vi "ReadDriveEncoder.vi"() -> ()   [LabVIEW 2012]
uses:
  Robot Global Data.vi
panel:
  out "EncoderR Alarm Status":string
  out "DistanceR (in)":dbl
  out "RevolutionsR":dbl
  out "Current angleR (deg)":dbl(knob) scale=0.0..360.0
  out "EncoderR Rate (deg/sec)":dbl
  out "EncoderR Direction":string
  in  "Reset EncoderR?":bool
  out "EncoderL Direction":string
  out "EncoderL Alarm Status":string
  in  "Reset EncoderL?":bool
  out "EncoderL Rate (deg/sec)":dbl
  out "RevolutionsL":dbl
  out "DistanceL (in)":dbl
  out "Current angleL (deg)":dbl(knob) scale=0.0..360.0
  out "error out":errorcluster
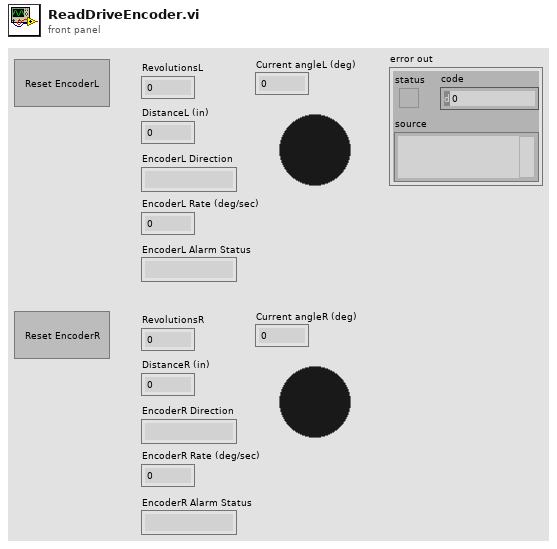
[diagram p1: front panel]
types:
  T1 = typedef "WPI_EncoderDevRef.ctl" = cluster{"DevStatus":errorcluster, "EncoderIndex":T2, "CounterIndex":T3, "DistancePerCount":dbl, "Decoding Type":T4}
  T2 = typedef "FPGA_EncoderIdx.ctl" = enum8{"Enc 0", "Enc 1", "Enc 2", "Enc 3", "Invalid"}
  T3 = typedef "FPGA_CounterCtrSystemIndex.ctl" = enum8{"Ctr 0", "Ctr 1", "Ctr 2", "Ctr 3", "Ctr 4", "Ctr 5", "Ctr 6", "Ctr 7", "Invalid"}
  T4 = typedef "WPI_EncoderType.ctl" = enum16{"1x", "2x", "4x"}
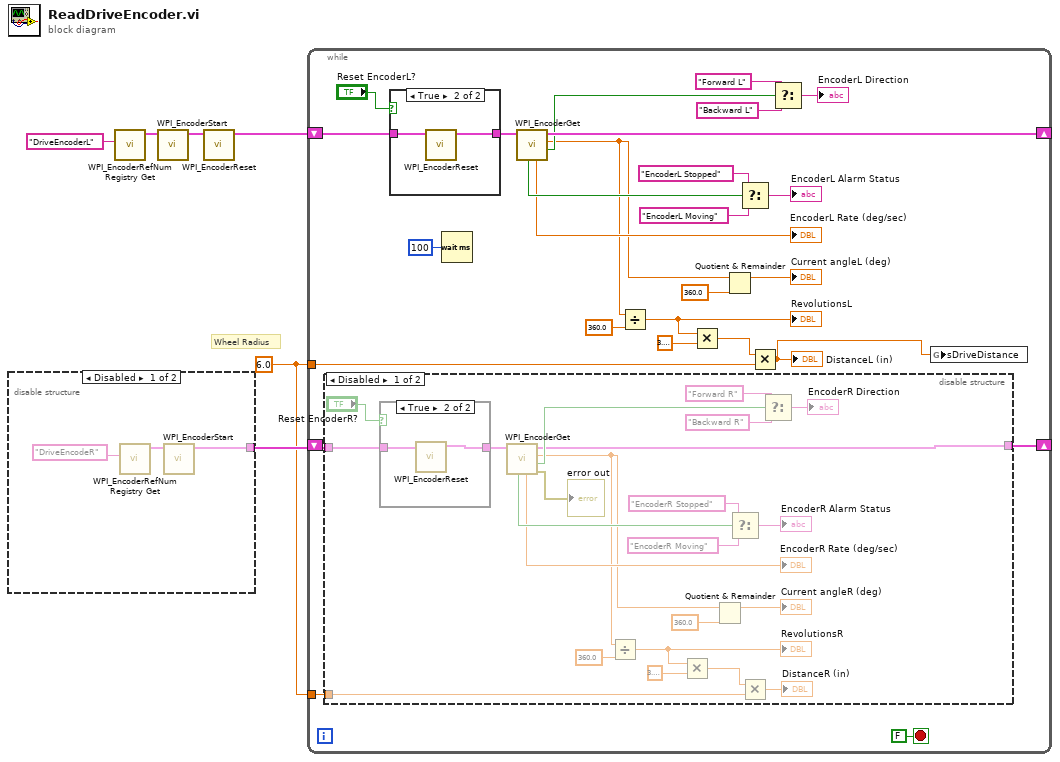
[diagram p0: block diagram]
diagram:
  w2 = 6.0
  # "Wheel Radius"
  n1 = disable-structure shown="Disabled" {
    disable-tunnel: [w7 _] -> w3
    frame Disabled {
      n2 = call <vilib>:"WPI_EncoderRefNum Registry Get.vi"("refnum name"="DriveEncodeR") -> ("EncoderDevRef"=w9:T1)  [unwired: 9 in, 1 out]
      n3 = call <vilib>:"WPI_EncoderStart.vi"("EncoderDevRef"=w9) -> ("EncoderDevRef"=w7:T1)  [unwired: 1 in, 9 out]
    }
    frame Enabled {
    }
  }
  n4 = call <vilib>:"WPI_EncoderRefNum Registry Get.vi"("refnum name"="DriveEncoderL") -> ("EncoderDevRef"=w6:T1)  [unwired: 9 in, 1 out]
  n5 = call <vilib>:"WPI_EncoderStart.vi"("EncoderDevRef"=w6) -> ("EncoderDevRef"=w5:T1)  [unwired: 1 in, 9 out]
  n6 = call <vilib>:"WPI_EncoderReset.vi"("EncoderDevRef"=w5) -> ("EncoderDevRef"=w1:T1)  [unwired: 1 in, 9 out]
  n7 = while {
    shift-right: [w32] -> _
    shift-left: w1 -> [w34]
    tunnel: w2 -> [w16]
    shift-right: [w14] -> _
    shift-left: w3 -> [w13]
    tunnel: w2 -> [w12]
    stop <- FALSE stop-if-true
    n8 = disable-structure shown="Disabled" {
      disable-tunnel: [w41 _] -> w14
      disable-tunnel: w13 -> [w40 _]
      disable-tunnel: w12 -> [w38 _]
      frame Disabled {
        n9 = case shown="True" "Reset EncoderR?" {
          tunnel: [w60 w62] -> w58
          tunnel: w40 -> [w60 w61]
          frame False {
          }
          frame True {
            n10 = call <vilib>:"WPI_EncoderReset.vi"("EncoderDevRef"=w61) -> ("EncoderDevRef"=w62:T1)  [unwired: 9 in, 1 out]
          }
        }
        n11 = call <vilib>:"WPI_EncoderGet.vi"("EncoderDevRef"=w58) -> ("error out"=→"error out":errorcluster, "Direction"=w54:bool, "Distance"=w37:dbl, "EncoderDevRef"=w41:T1, "Rate"=→"EncoderR Rate (deg/sec)":dbl, "Stopped"=w51:bool)  [unwired: 5 in]
        n12 = Divide(x=w37, y=360.0) -> (x/y=w44:dbl)
        "RevolutionsR" <- w44
        n13 = Multiply(x=w44, y=3.141592653589793) -> (x*y=w42:dbl)
        n14 = Quotient & Remainder(x=w37, y=360.0) -> (x-y*floor(x/y)=→"Current angleR (deg)":dbl)  [unwired: 1 out]
        n15 = Select(t="EncoderR Stopped", s=w51, f="EncoderR Moving") -> (s? t:f=→"EncoderR Alarm Status":string)
        n16 = Multiply(x=w42, y=w38) -> (x*y=→"DistanceR (in)":dbl)
        n17 = Select(t="Forward R", s=w54, f="Backward R") -> (s? t:f=→"EncoderR Direction":string)
      }
      frame Enabled {
      }
    }
    n18 = case shown="True" "Reset EncoderL?" {
      tunnel: w34 -> [w63 w65]
      tunnel: [w63 w64] -> w33
      frame False {
      }
      frame True {
        n19 = call <vilib>:"WPI_EncoderReset.vi"("EncoderDevRef"=w65) -> ("EncoderDevRef"=w64:T1)  [unwired: 9 in, 1 out]
      }
    }
    n20 = Wait (ms)(milliseconds to wait=u32 100) -> ()  [unwired: 1 out]
    n21 = call <vilib>:"WPI_EncoderGet.vi"("EncoderDevRef"=w33) -> ("Direction"=w28:bool, "Distance"=w11:dbl, "EncoderDevRef"=w32:T1, "Rate"=→"EncoderL Rate (deg/sec)":dbl, "Stopped"=w25:bool)  [unwired: 5 in, 1 out]
    n22 = Divide(x=w11, y=360.0) -> (x/y=w18:dbl)
    "RevolutionsL" <- w18
    n23 = Multiply(x=w18, y=3.141592653589793) -> (x*y=w17:dbl)
    n24 = Quotient & Remainder(x=w11, y=360.0) -> (x-y*floor(x/y)=→"Current angleL (deg)":dbl)  [unwired: 1 out]
    n25 = Select(t="EncoderL Stopped", s=w25, f="EncoderL Moving") -> (s? t:f=→"EncoderL Alarm Status":string)
    n26 = Multiply(x=w17, y=w16) -> (x*y=w10:dbl)
    "DistanceL (in)" <- w10
    n27 = Select(t="Forward L", s=w28, f="Backward L") -> (s? t:f=→"EncoderL Direction":string)
    n28 = global write "Robot Global Data.vi" "sDriveDistance"(w10) -> ()
  }
